vi "Looper_str.vi"(9 "Num Points":string, 10 "Max":string, 11 "Min":string) -> (1 "Result":dbl[](array[numeric]), 2 "Result (str)":string[](array[string]))   [LabVIEW 2018]
panel:
  out "Delta":dbl
  out "Step Size":dbl
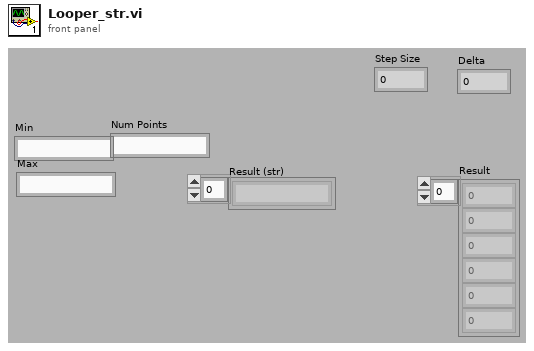
[diagram p1: front panel]
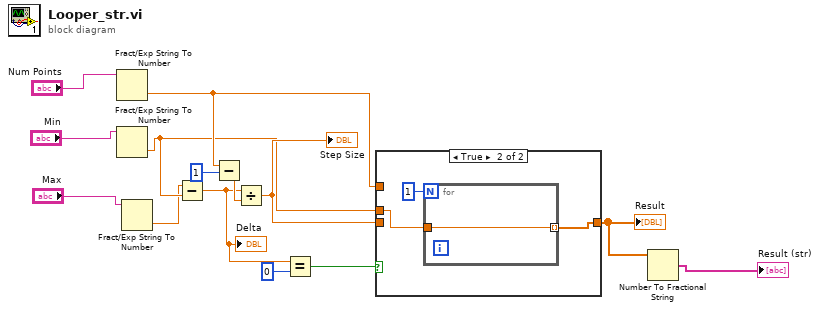
[diagram p0: block diagram]
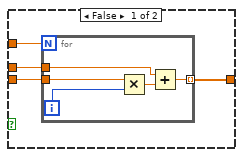
[diagram p2: hidden frame]
diagram:
  n1 = Fract/Exp String To Number(string="Num Points") -> (number=w6:dbl)  [unwired: 3 in, 1 out]
  n2 = Fract/Exp String To Number(string="Min") -> (number=w4:dbl)  [unwired: 3 in, 1 out]
  n3 = Fract/Exp String To Number(string="Max") -> (number=w1:dbl)  [unwired: 3 in, 1 out]
  n4 = Subtract(x=w1, y=w4) -> (x-y=w11:dbl)
  "Delta" <- w11
  n5 = Subtract(x=w6, y=1) -> (x-y=w13:dbl)
  n6 = Divide(x=w11, y=w13) -> (x/y=w14:dbl)
  "Step Size" <- w14
  n7 = Equal?(x=w11, y=0) -> (x = y?=w9:bool)
  n8 = case shown="True" w9 {
    tunnel: w14 -> [w18 _]
    tunnel: w4 -> [w17 w24]
    tunnel: w6 -> [w16 _]
    tunnel: [w15 w26] -> w8
    frame False {
      n9 = for {
        N: w16 -> [_]
        tunnel: w17 -> [w20]
        tunnel: w18 -> [w22]
        tunnel: [w19] -> w15 mode=indexing
        i -> [w23]
        n10 = Multiply(x=w22, y=w23) -> (x*y=w21:dbl)
        n11 = Add(x=w20, y=w21) -> (x+y=w19:dbl)
      }
    }
    frame True {
      n12 = for {
        N: 1 -> [_]
        tunnel: [w27] -> w26 mode=indexing
        tunnel: w24 -> [w27]
      }
    }
  }
  "Result" <- w8
  n13 = Number To Fractional String(number=w8) -> (F-format string=→"Result (str)":string[])  [unwired: 3 in]
